vi "GT Get Count Config.vi"(7 "pCount":T1, 8 "error in (no error)":errorcluster caption="错误输入（无错误）", 9 "countIndex":i16, 10 "countType":i16, 11 "cardNum":i16) -> (0 "error out":errorcluster caption="错误输出", 3 "function return":i16, 5 "pCount out":T1)   [LabVIEW 2020, in "gts1.lvlib"]
doc: "GT_API GT_GetCountConfig(short cardNum,short countType,short countIndex,TCountConfig *pCount);"
uses:
  gts1.lvlib
  dll/32bit/multi_card/gts.dll
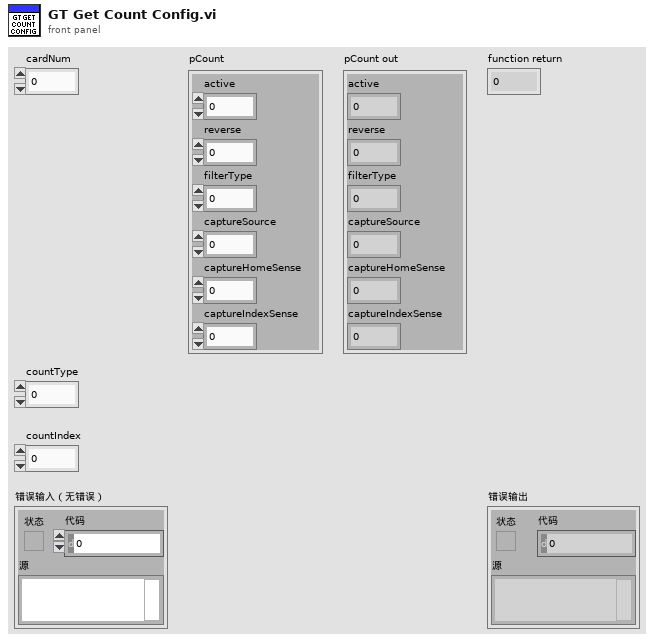
[diagram p1: front panel]
types:
  T1 = cluster{"active":i16, "reverse":i16, "filterType":i16, "captureSource":i16, "captureHomeSense":i16, "captureIndexSense":i16}
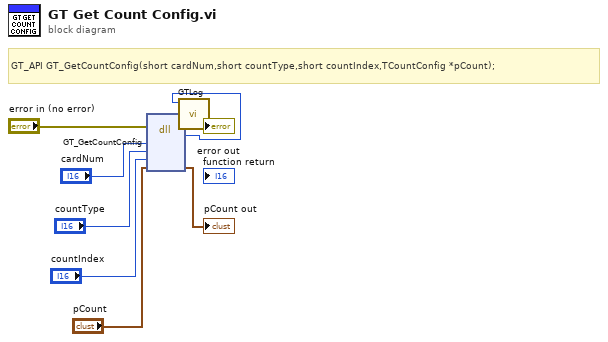
[diagram p0: block diagram]
diagram:
  # "GT_API GT_GetCountConfig(short cardNum,short countType,short countIndex,TCountConfig *pCount);"
  n1 = dll-call lib="C:/1228/dll/32bit/multi_card/gts.dll" fn="GT_GetCountConfig"(error in="error in (no error)", "cardNum"="cardNum", "countType"="countType", "countIndex"="countIndex", "pCount"="pCount") -> (error out=w3:errorcluster, w1:i16, "pCount"=→"pCount out":T1)  [unwired: 5 in, 1 out]
  n2 = call "GTLog.vi"("error in (no error)"=w3, "Numeric"=w1) -> ("error out"=→"error out":errorcluster)  [unwired: 9 in]
